vi "Reset.vi"(8 "error in":errorcluster, 11 "VISA resource name":refnum<visa-resource-name>) -> (0 "error out":errorcluster, 3 "VISA resource out":refnum<visa-resource-name>)   [LabVIEW 2019, in "Acopian.lvlib" / "Acopian.lvclass"]
uses:
  Library/Acopian.lvclass
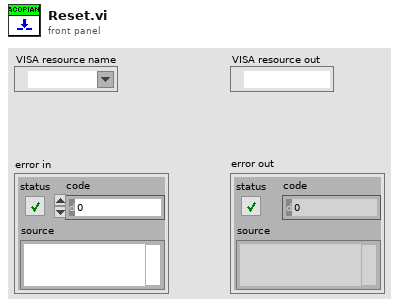
[diagram p1: front panel]
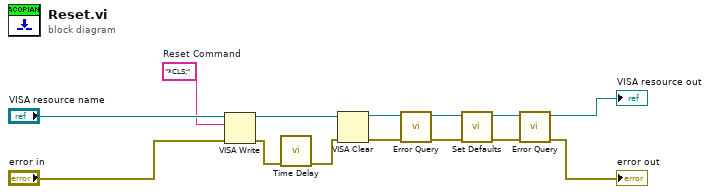
[diagram p0: block diagram]
diagram:
  w7 = "*CLS;"  # Reset Command
  n1 = VISA Write(VISA resource name="VISA resource name", write buffer=w7, error in (no error)="error in") -> (VISA resource name out=w8:refnum<visa-resource-name>, error out=w10:errorcluster)  [unwired: 1 out]
  n2 = call "Time Delay"("error in (no error)"=w10) -> ("error out"=w9:errorcluster)  [unwired: 10 in]
  n3 = VISA Clear(VISA resource name=w8, error in (no error)=w9) -> (VISA resource name out=w6:refnum<visa-resource-name>, error out=w5:errorcluster)
  n4 = call "Error Query.vi"("error in"=w5, "VISA resource in"=w6) -> ("error out"=w4:errorcluster, "VISA resource out"=w3:refnum<visa-resource-name>)  [unwired: 6 in, 2 out]
  n5 = call "Set Defaults.vi"("error in"=w4, "VISA resource name"=w3) -> ("error out"=w2:errorcluster, "VISA resource name out"=w1:refnum<visa-resource-name>)  [unwired: 8 in]
  n6 = call "Error Query.vi"("error in"=w2, "VISA resource in"=w1) -> ("error out"=→"error out":errorcluster, "VISA resource out"=→"VISA resource out":refnum<visa-resource-name>)  [unwired: 6 in, 2 out]
